vi "TTC001ConnectSetDisplayTemp.vi"() -> ()   [LabVIEW 2023]
uses:
  C:/Users/fmovagharnemati/OneDrive - THORLABS Inc/Desktop/github/KPC101/Thorlabs.MotionControl.Controls.dll
  github/KPC101/Thorlabs.MotionControl.Controls.dll
  C:/Users/fmovagharnemati/OneDrive - THORLABS Inc/Desktop/github/KPC101/Thorlabs.MotionControl.TCube.TECCLI.dll
  github/KPC101/Thorlabs.MotionControl.TCube.TECCLI.dll
panel:
  out "temperature/resistance reading":dbl
  in  "Disconnect":bool
  in  "Set Temp":bool
  in  "Set Point":dbl
  in  "SerialNumber":string
  in  "TCubeTECControl":refnum<k24>(container)
  # "Thorlabs Hardware: TTC001 - T-Cube TEC Controller\nhttps://www.thorlabs.com/thorproduct.cfm?partnumber=TTC001\n\nDescription: This VI will enable you to communicate with TTC001 to set a desired temperature and get live readings of current temperature. The VI will first connect and initialize the device, and waits for user command for the temperature set point.\n\nInstructions: \n1) Connect your TTC001 device to your PC & power the device, ensuring your TEC is connected. For full device setup, the device product manual can be found on our website here. -https://www.thorlabs.com/thorproduct.cfm?partnumber=TTC001\n2) Enter the device serial number below.\n3) Click 'Run' in the LabVIEW Toolbar which will attempt a connection.\n4) Await for device to be be available.\n5) Input desired temperature, and press 'Set Temp'.\n6) To end the Program click 'STOP'."
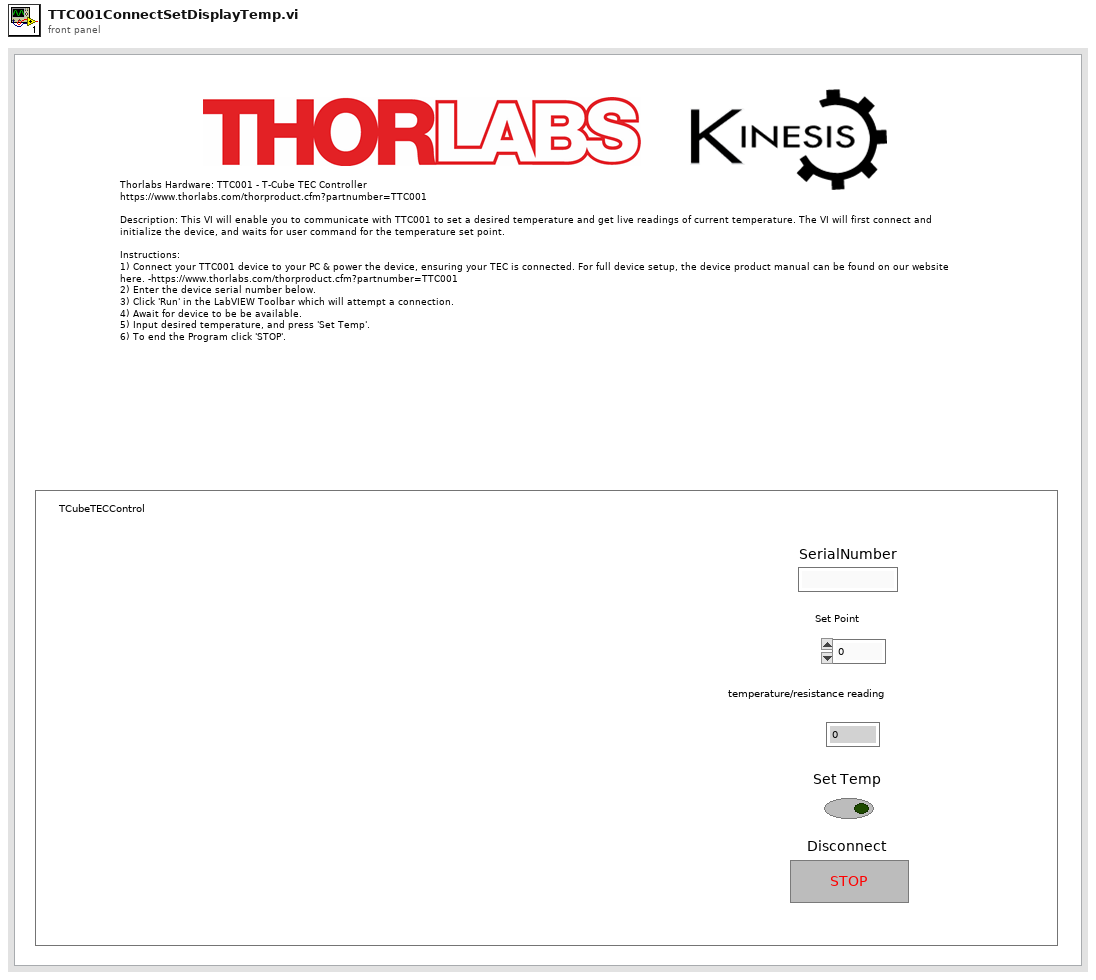
[diagram p1: front panel]
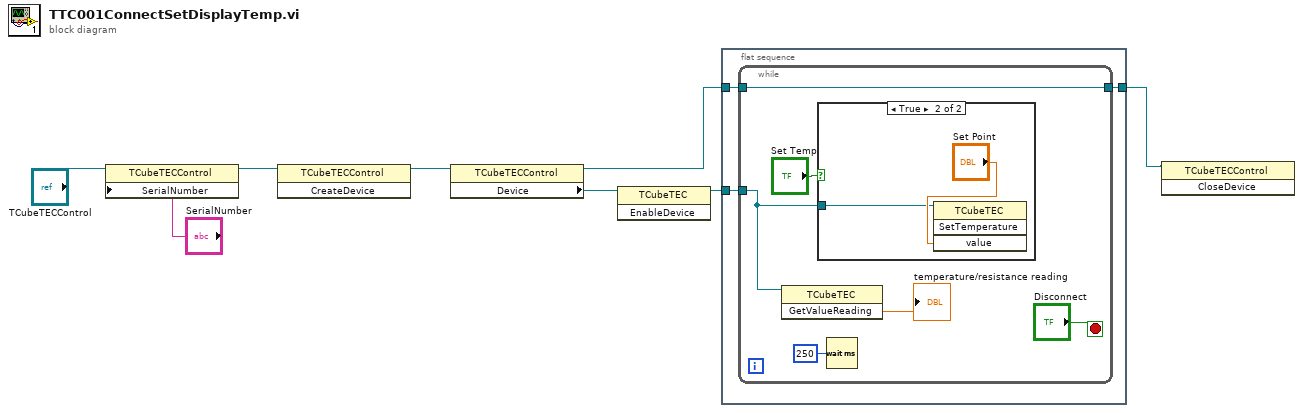
[diagram p0: block diagram]
diagram:
  n1 = property class="TCubeTECControl"(reference="TCubeTECControl", "SerialNumber"="SerialNumber") -> (reference out=w7:refnum<k24>)  [unwired: 1 in, 1 out]
  n2 = invoke class="TCubeTECControl" method="CreateDevice"(reference=w7) -> (reference out=w6:refnum<k24>)  [unwired: 2 in, 2 out]
  n3 = property class="TCubeTECControl"(reference=w6) -> (reference out=w4:refnum<k24>, "Device"=w5:refnum<k24>)  [unwired: 1 in, 1 out]
  n4 = invoke class="TCubeTEC" method="EnableDevice"(reference=w5) -> (reference out=w2:refnum<k24>)  [unwired: 2 in, 2 out]
  n5 = flat-sequence {
    tunnel: [w11] -> w3
    tunnel: w4 -> [w10]
    tunnel: w2 -> [w9]
    frame #0 {
      n6 = while {
        tunnel: [w13] -> w11
        tunnel: w10 -> [w13]
        tunnel: w9 -> [w12]
        stop <- "Disconnect" stop-if-true
        n7 = invoke class="TCubeTEC" method="GetValueReading"(reference=w12) -> ("GetValueReading"=→"temperature/resistance reading":dbl)  [unwired: 2 in, 2 out]
        n8 = case shown="True" "Set Temp" {
          tunnel: w12 -> [_ w18]
          frame False {
          }
          frame True {
            n9 = invoke class="TCubeTEC" method="SetTemperature"(reference=w18, "value"="Set Point") -> ()  [unwired: 2 in, 4 out]
          }
        }
        n10 = Wait (ms)(milliseconds to wait=u32 250) -> ()  [unwired: 1 out]
      }
    }
  }
  n11 = invoke class="TCubeTECControl" method="CloseDevice"(reference=w3) -> ()  [unwired: 2 in, 3 out]
